vi "_Format Memory Map String.vi"(4 "User value":string, 5 "Data":i32, 6 "Address":u16, 7 "String In":string) -> (3 "String Out":string)   [LabVIEW 2015]
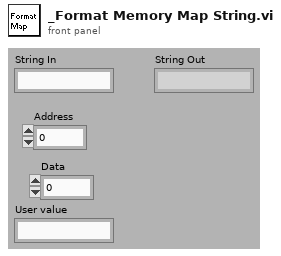
[diagram p1: front panel]
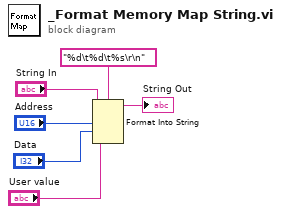
[diagram p0: block diagram]
diagram:
  n1 = Format Into String(format string="%d\t%d\t%s\r\n", initial string="String In", "Address", "Data", "User value") -> (resulting string=→"String Out":string)  [unwired: 1 in, 1 out]
